vi "ConfigureTrigger.vi"(8 "error in (no error)":errorcluster, 9 "Simulation":T2, 10 "Trigger":T3={"Level"=0.04, "Source"=enum."Channel 2", "Slope"=enum."Rising", "mode"=enum."Single", "Autotrigger"=0.04} {"Autotrigger" format="%#_6p"; "Level" format="%#_6p"}, 11 "picoscope in":refnum<class "picoscope.lvclass">) -> (0 "error out":errorcluster, 2 "Trigger":T3={"Level"=0.04, "Source"=enum."Channel 2", "Slope"=enum."Rising", "mode"=enum."Single", "Autotrigger"=0.04} {"Autotrigger" format="%#_6p"; "Level" format="%#_6p"}, 3 "picoscope out":refnum<class "picoscope.lvclass">)   [LabVIEW 2020, in "picoscope.lvclass"]
uses:
  picoscope.lvclass
  LeCroy Sub VI's/trigger ctl.ctl
  shared/OnOffTypeDef.ctl
  picoscope.lvclass/picoscope.ctl
panel:
  out "Trigger Settings":T1={"Trigger Enabled"=FALSE, "Trigger Source"=enum."Channel A", "Trigger Threshold (volts)"=0.0, "Trigger Direction"=2, "Trigger Delay (samples)"=0, "Auto Trigger Time (ms)"=1000} {"Trigger Direction" items=["Rising"=2, "Falling"=3]}
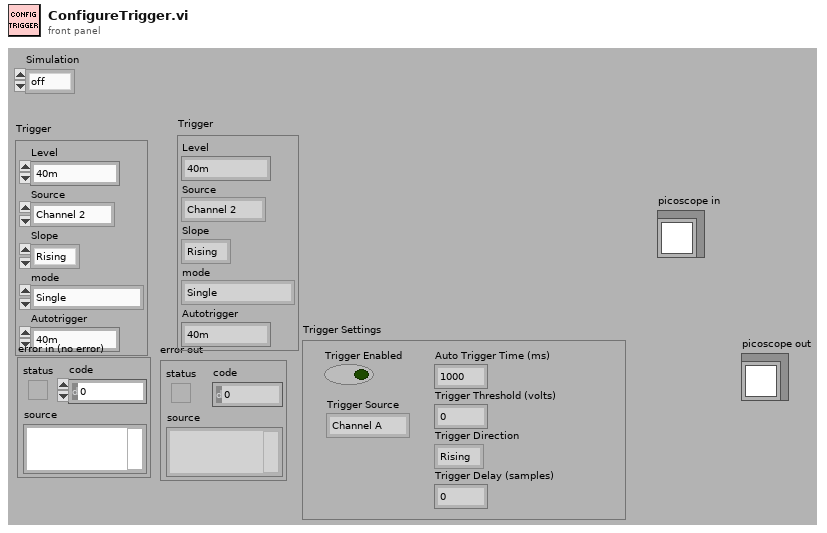
[diagram p1: front panel]
types:
  T1 = cluster{"Trigger Enabled":bool, "Trigger Source":enum16{"Channel A", "Channel B", "Channel C", "Channel D", "Ext."}, "Trigger Threshold (volts)":dbl, "Trigger Direction":u16, "Trigger Delay (samples)":u32, "Auto Trigger Time (ms)":i16}
  T2 = typedef "OnOffTypeDef.ctl" = enum16{"off", "on"}
  T3 = typedef "trigger ctl.ctl" = cluster{"Level":dbl, "Source":enum16{"Channel 1", "Channel 2", "Channel 3", "Channel 4", "External", "Power Line"}, "Slope":enum16{"Rising", "Falling"}, "mode":enum16{"Auto", "Normal", "Single", "Single auto trigger"}, "Autotrigger":dbl}
  T4 = enum16{"Channel A", "Channel B", "Channel C", "Channel D", "Ext."}
  T5 = enum16{"Channel 1", "Channel 2", "Channel 3", "Channel 4", "External", "Power Line"}
  T6 = enum16{"Auto", "Normal", "Single", "Single auto trigger"}
  T7 = cluster{"Enabled":bool, "Coupling":i16, "Range":u16, "Analogue Offset":sgl}
  T8 = cluster{"Driver Version":string, "USB Version":string, "Hardware":string, "Variant":string, "Batch and Serial":string, "Cal Date":string, "Kernel Version":string, "Digital HW Version":string, "Analogue HW Version":string, "MSO":bool, "Number of channels":i16}
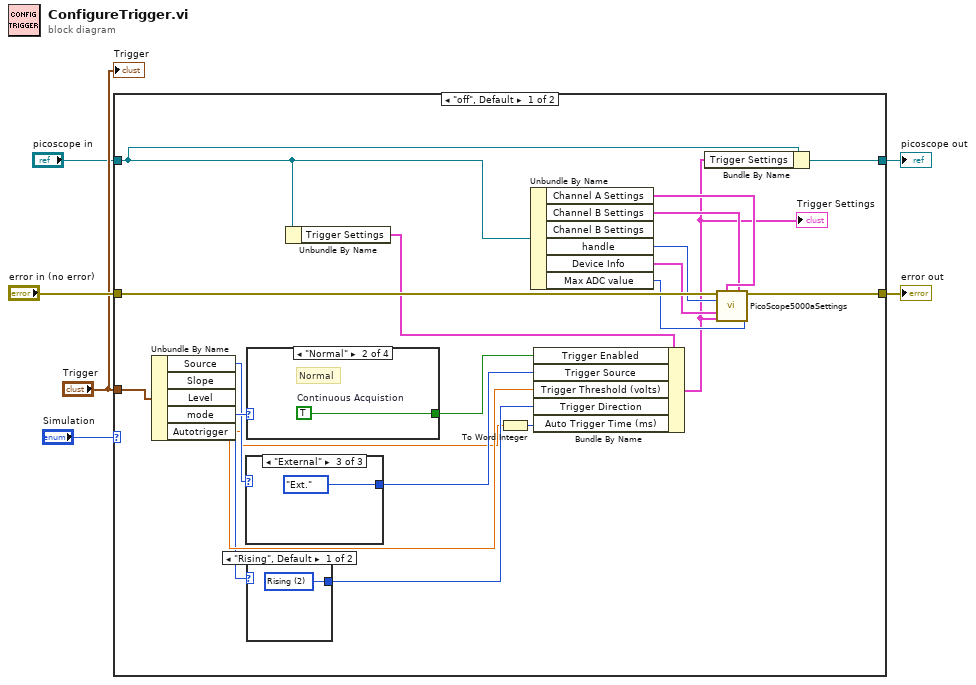
[diagram p0: block diagram]
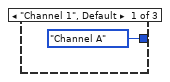
[diagram p2: hidden frame]
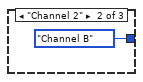
[diagram p3: hidden frame]
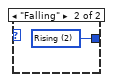
[diagram p4: hidden frame]
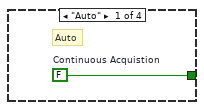
[diagram p5: hidden frame]
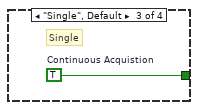
[diagram p6: hidden frame]
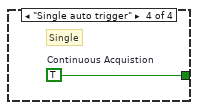
[diagram p7: hidden frame]
diagram:
  n1 = case shown="\"off\", Default" "Simulation" {
    tunnel: [w20 w38] -> w6
    tunnel: "Trigger" -> [w26 _]
    tunnel: "error in (no error)" -> [w19 w38]
    tunnel: "picoscope in" -> [w10 w37]
    tunnel: [w21 w37] -> w1
    frame "off", Default {
      n2 = Unbundle By Name(w26) -> ("Source"=w13:T5, "Slope"=w15:enum16{"Rising", "Falling"}, "Level"=w22:dbl, "mode"=w27:T6, "Autotrigger"=w7:dbl)
      n3 = case shown="\"External\"" w13 {
        tunnel: [T4."Channel A" ("Trigger Source") T4."Channel B" ("Trigger Source") T4."Ext." ("Trigger Source")] -> w12
        frame "Channel 1", Default {
        }
        frame "Channel 2" {
        }
        frame "External" {
        }
      }
      n4 = case shown="\"Normal\"" w27 {
        tunnel: [w33 w34 w35 w36] -> w23
        frame "Auto" {
          w33 = FALSE  # Continuous Acquistion
          # "Auto"
        }
        frame "Normal" {
          w34 = TRUE  # Continuous Acquistion
          # "Normal"
        }
        frame "Single", Default {
          w35 = TRUE  # Continuous Acquistion
          # "Single"
        }
        frame "Single auto trigger" {
          w36 = TRUE  # Continuous Acquistion
          # "Single"
        }
      }
      n5 = case shown="\"Rising\", Default" w15 {
        tunnel: [w31 w32] -> w14
        frame "Rising", Default {
          w31 = u16 2 items=["Rising"=2, "Falling"=3] ("Trigger Direction")
        }
        frame "Falling" {
          w32 = u16 2 items=["Rising"=2, "Falling"=3] ("Trigger Direction")
        }
      }
      n6 = Unbundle By Name(w10) -> ("Trigger Settings"=w9:T1)
      n7 = To Word Integer(number=w7) -> (16bit integer=w8:i16)
      n8 = Unbundle By Name(w10) -> ("Channel A Settings"=w25:T7, "Channel B Settings"=w24:T7, "handle"=w18:i16, "Device Info"=w17:T8, "Max ADC value"=w16:i16)  [unwired: 1 out]
      n9 = Bundle By Name(cluster=w9, "Trigger Enabled"=w23, "Trigger Source"=w12, "Trigger Threshold (volts)"=w22, "Trigger Direction"=w14, "Auto Trigger Time (ms)"=w8) -> (w11:T1)
      "Trigger Settings" <- w11
      n10 = Bundle By Name(cluster=w10, "Trigger Settings"=w11) -> (w21:refnum<class "picoscope.lvclass">)
      n11 = call "PicoScope5000aSettings.vi"("error in"=w19, "Channel A Settings"=w25, "Channel B Settings"=w24, "handle in"=w18, "Device Info"=w17, "Trigger Settings"=w11, "Max ADC value"=w16) -> ("error out"=w20:errorcluster)  [unwired: 6 in, 2 out]
    }
    frame "on" {
      # "Simulation Mode ON"
    }
  }
  "error out" <- w6
  "picoscope out" <- w1
  "Trigger" <- "Trigger"
